vi "AlliGator Decode PI Imaging Metadata Field.vi"(11 "Metadata Text Field":string) -> (1 "Metadata":string, 2 "Field":string)   [LabVIEW 2021, in "AlliGator Files.lvlib"]
doc: "Extract metadata from a Pi Imaging gate image field."
uses:
  <vilib>/Utility/error.llb/Error Cluster From Error Code.vi
  <vilib>/ErrorRing/Error Ring.xnode
  AlliGator Files.lvlib
panel:
  out "Error Out":errorcluster
  in  "Error In":errorcluster
  # "see the AlliGator License on the block diagram (Ctrl+E or Window:Show Block Diagram)"
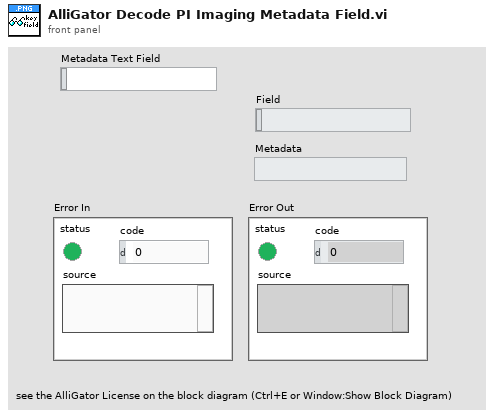
[diagram p1: front panel]
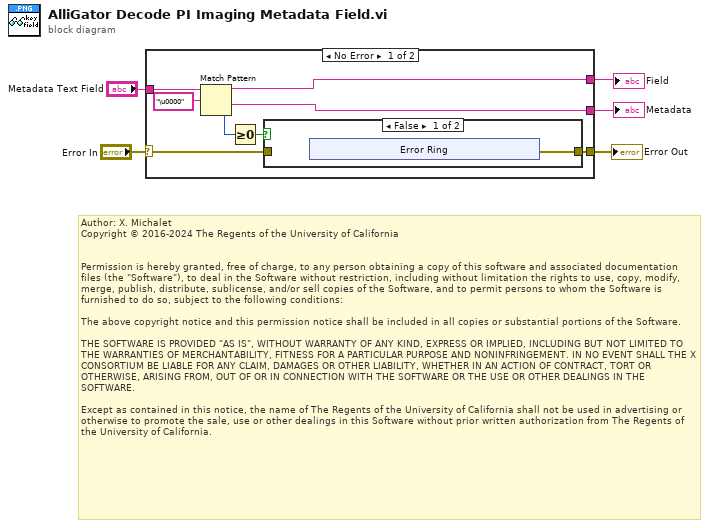
[diagram p0: block diagram]
diagram:
  # "Author: X. Michalet\nCopyright © 2016-2024 The Regents of the University of California\n \n\nPermission is hereby granted, free of charge, to any person obtaining a copy of this software and associated documentation files (the \"Software\"), to deal in the Software without restriction, including without limitation the rights to use, copy, modify, merge, publish, distribute, sublicense, and/or sell copies of the Software, and to permit persons to whom the Software is furnished to do so, subject to the following conditions:\n\nThe above copyright notice and this permission notice shall be included in all copies or substantial portions of the Software.\n\nTHE SOFTWARE IS PROVIDED \"AS IS\", WITHOUT WARRANTY OF ANY KIND, EXPRESS OR IMPLIED, INCLUDING BUT NOT LIMITED TO THE WARRANTIES OF MERCHANTABILITY, FITNESS FOR A PARTICULAR PURPOSE AND NONINFRINGEMENT. IN NO EVENT SHALL THE X CONSORTIUM BE LIABLE FOR ANY CLAIM, DAMAGES OR OTHER LIABILITY, WHETHER IN AN ACTION OF CONTRACT, TORT OR OTHERWISE, ARISING FROM, OUT OF OR IN CONNECTION WITH THE SOFTWARE OR THE USE OR OTHER DEALINGS IN THE SOFTWARE.\n\nExcept as contained in this notice, the name of The Regents of the University of California shall not be used in advertising or otherwise to promote the sale, use or other dealings in this Software without prior written authorization from The Regents of the University of California."
  n1 = case shown="No Error" "Error In" {
    selector: "Error In" -> [w7 w20]
    tunnel: [w13 _] -> w5
    tunnel: "Metadata Text Field" -> [w12 _]
    tunnel: [w9 _] -> w3
    tunnel: [w6 w20] -> w1
    frame No Error {
      n2 = Match Pattern(string=w12, regular expression="\u0000" ("String")) -> (before substring=w9:string, after substring=w13:string, offset past match=w10:i32)  [unwired: 1 in, 1 out]
      n3 = Greater Or Equal To 0?(x=w10) -> (x >= 0?=w8:bool)
      n4 = case shown="False" w8 {
        tunnel: w7 -> [_ w19]
        tunnel: [w14 w19] -> w6
        frame False {
          n5 = xnode "Error Ring"() -> ("error out"=w14:errorcluster)
        }
        frame True {
        }
      }
    }
    frame Error {
    }
  }
  "Metadata" <- w5
  "Field" <- w3
  "Error Out" <- w1
